vi "save data.vi"(9 "name":string, 10 "Path":path, 11 "cluster":cluster{"T&Y(output)":dbl[][], "dt":dbl} {"dt" format="%#_13g"}) -> (1 "path (for gaussian":path, 2 "new file path (Not A Path if cancelled)":path, 3 "path(FOR logistic":path)   [LabVIEW 2018]
uses:
  <vilib>/Utility/file.llb/Write Delimited Spreadsheet (DBL).vi
panel:
  out "concatenated string":string
  out "file name(row data)":string
  out "file name":string
  in  "time stamp":timestamp format="%<%H:%M:%S\n%m/%d/%Y>T"
  out "slope":dbl[](array[numeric])
  out "dt":dbl
  out "y":dbl[](array[numeric])
  out "t":dbl[](array[numeric])
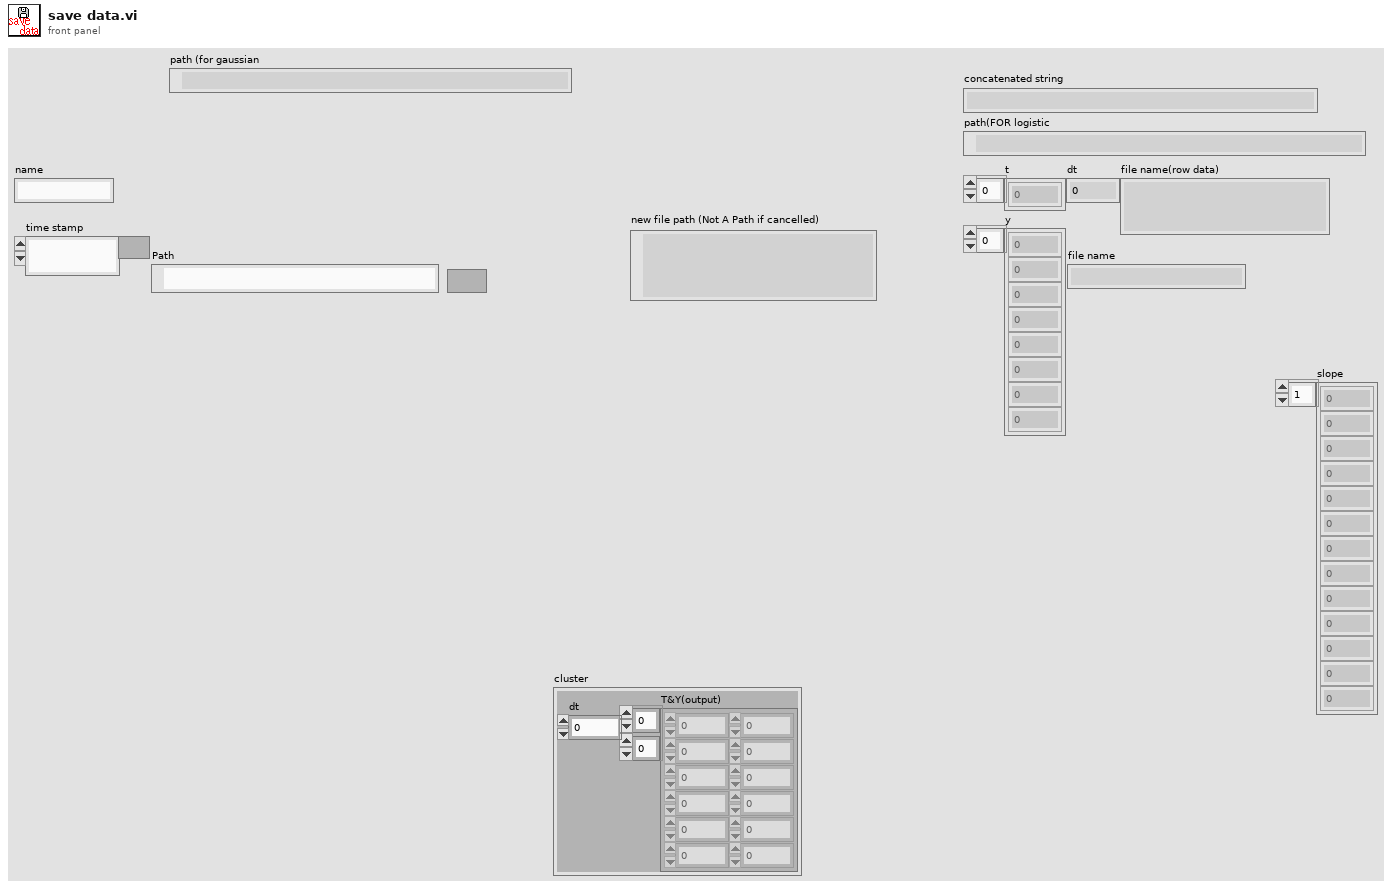
[diagram p1: front panel]
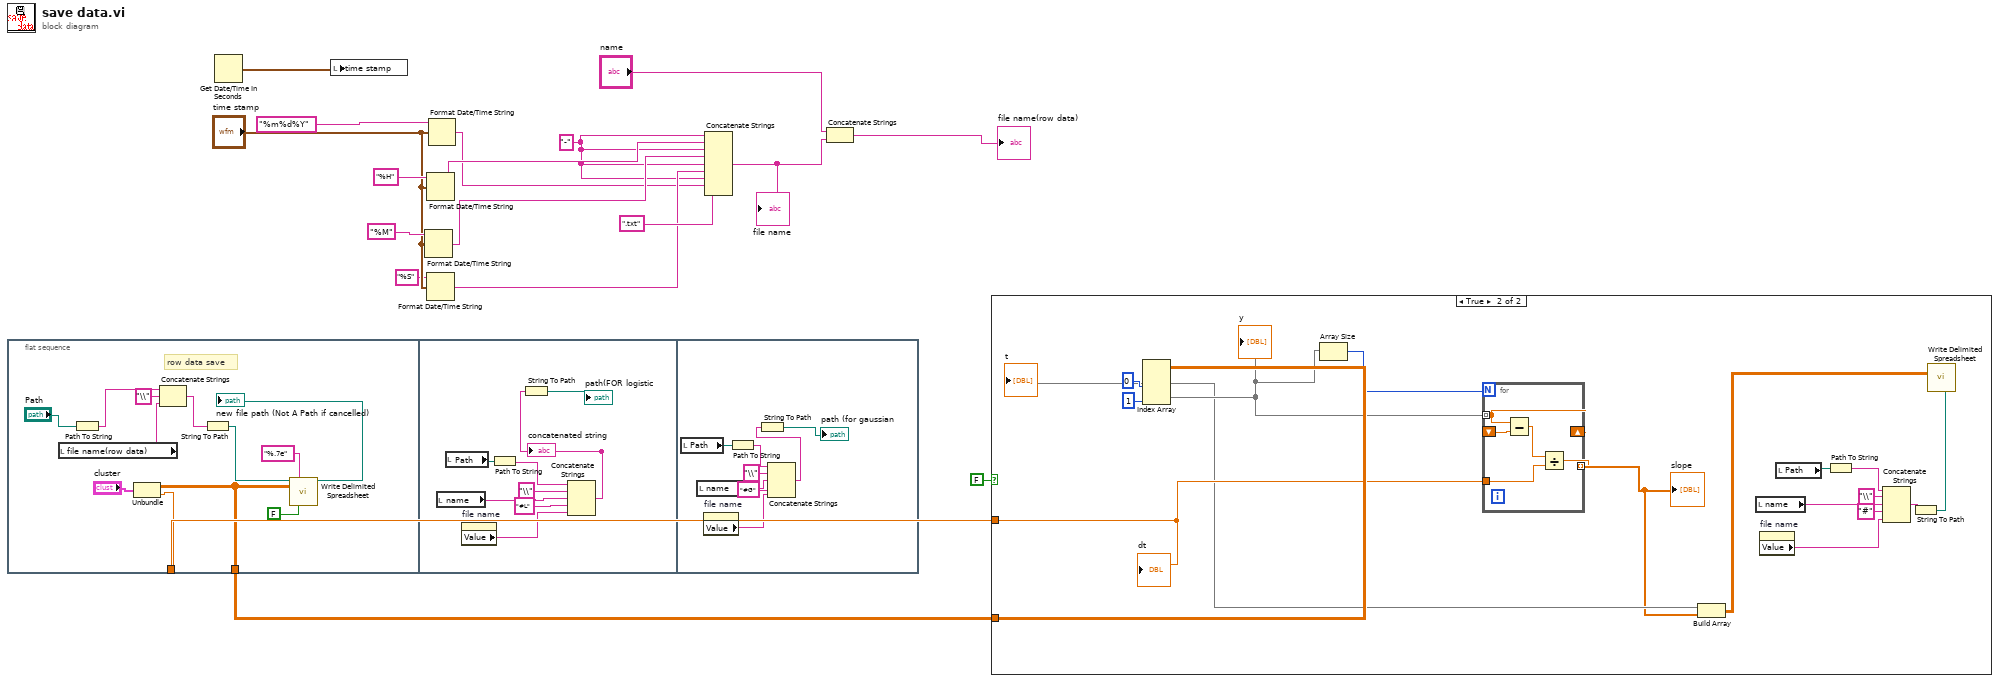
[diagram p0: block diagram]
diagram:
  w4 = "-" ("string")
  n1 = flat-sequence {
    tunnel: [w26] -> w17
    tunnel: [w25] -> w18
    frame #0 {
      # "row data save"
      n2 = local read "file name(row data)"() -> (w22:string)
      n3 = Path To String(path="Path") -> (string=w24:string)
      n4 = Unbundle("cluster") -> ("T&Y(output)"=w25:dbl[][], "dt"=w26:dbl)
      n5 = Concatenate Strings(w24, "\\" ("string"), w22) -> (w21:string)
      n6 = String To Path(string=w21) -> (path=w20:path)
      n7 = call-poly <vilib>:"Write Delimited Spreadsheet.vi"("file path (dialog if empty)"=w20, "format (%.3f)"="%.7e", "2D data"=w25, "transpose? (no:F)"=FALSE) -> ("new file path (Not A Path if cancelled)"=→"new file path (Not A Path if cancelled)":path)  [unwired: 10 in, 1 out]
    }
    frame #1 {
      n8 = local read "name"() -> (w34:string)
      n9 = local read "Path"() -> (w35:path)
      n10 = property on="file name" class="Str"() -> ("Value"=w33:string)  [unwired: 2 in, 2 out]
      n11 = Path To String(path=w35) -> (string=w36:string)
      n12 = Concatenate Strings(w36, "\\" ("string"), w34, "#L" ("string"), w33) -> (w31:string)
      "concatenated string" <- w31
      n13 = String To Path(string=w31) -> (path=→"path(FOR logistic":path)
    }
    frame #2 {
      n14 = local read "Path"() -> (w43:path)
      n15 = local read "name"() -> (w45:string)
      n16 = property on="file name" class="Str"() -> ("Value"=w40:string)  [unwired: 2 in, 2 out]
      n17 = Path To String(path=w43) -> (string=w44:string)
      n18 = Concatenate Strings(w44, "\\" ("string"), w45, "#G" ("string"), w40) -> (w46:string)
      n19 = String To Path(string=w46) -> (path=→"path (for gaussian":path)
    }
  }
  n20 = Get Date/Time In Seconds() -> (seconds since 1Jan1904=w16:timestamp)
  n21 = local write "time stamp"(w16) -> ()
  n22 = Format Date/Time String(time format string (%c)="%M", seconds (now)="time stamp") -> (date/time string=w6:string)  [unwired: 1 in]
  n23 = Format Date/Time String(time format string (%c)="%H", seconds (now)="time stamp") -> (date/time string=w7:string)  [unwired: 1 in]
  n24 = Format Date/Time String(time format string (%c)="%S", seconds (now)="time stamp") -> (date/time string=w5:string)  [unwired: 1 in]
  n25 = Format Date/Time String(time format string (%c)="%m%d%Y", seconds (now)="time stamp") -> (date/time string=w3:string)  [unwired: 1 in]
  n26 = Concatenate Strings(w4, w7, w4, w6, w4, w5, w4, w3, ".txt" ("string")) -> (w11:string)
  "file name" <- w11
  n27 = Concatenate Strings("name", w11) -> (→"file name(row data)":string)
  n28 = case shown="True" FALSE {
    tunnel: w18 -> [_ w63]
    tunnel: w17 -> [_ w60]
    frame False {
    }
    frame True {
      n29 = Index Array(array=w63, index (col) #1=0 ("disabled index (col)"), index (col) #2=1 ("index (col)")) -> (element #1=w57:dbl[], element #2=w59:dbl[])  [unwired: 2 in]
      "t" <- w57
      "y" <- w59
      n30 = Array Size(array=w59) -> (size(s)=w58:i32)
      n31 = for {
        N: w58 -> [_]
        shift-right: [w64] -> _
        shift-left: _ -> [w68]
        tunnel: w59 -> [w64] mode=indexing
        tunnel: w60 -> [w66]
        tunnel: [w65] -> w56 mode=indexing
        n32 = Subtract(x=w64, y=w68) -> (x-y=w67:dbl)
        n33 = Divide(x=w67, y=w66) -> (x/y=w65:dbl)
      }
      "slope" <- w56
      n34 = Build Array(w57, w56) -> (w55:dbl[][])
      n35 = local read "name"() -> (w54:string)
      n36 = property on="file name" class="Str"() -> ("Value"=w47:string)  [unwired: 2 in, 2 out]
      n37 = local read "Path"() -> (w48:path)
      n38 = Path To String(path=w48) -> (string=w49:string)
      n39 = Concatenate Strings(w49, "\\" ("string"), w54, "#" ("string"), w47) -> (w52:string)
      n40 = String To Path(string=w52) -> (path=w51:path)
      n41 = call-poly <vilib>:"Write Delimited Spreadsheet.vi"("file path (dialog if empty)"=w51, "2D data"=w55) -> ()  [unwired: 12 in, 2 out]
      "dt" <- w60
    }
  }
